vi "Distance PWM-Read.vi"(8 "Error":errorcluster, 11 "SonarMB1010DigitalDevRef":T1={"CounterDevRef"={"DevStatus"={"status"=FALSE, "code"=0, "source"=""}, "CntIndex"=enum."Invalid"}, "Min Distance"=0.000147, "Max Distance"=0.000147, "PWM Frequency"=0.0, "DIO Channel"=enum."DIO 0"}) -> (0 "Error Out":errorcluster, 2 "Distance Out":dbl, 3 "SonarMB1010DigitalDevRef Out":T1={"CounterDevRef"={"DevStatus"={"status"=FALSE, "code"=0, "source"=""}, "CntIndex"=enum."Invalid"}, "Min Distance"=0.000147, "Max Distance"=0.000147, "PWM Frequency"=0.0, "DIO Channel"=enum."DIO 0"})   [LabVIEW 2017]
doc: "Returns the distance, in inches, between the ultrasonic sensor and the closest object in front of the sensor. The ultrasonic sensor measures this distance by emitting a ping and calculating the time it takes for the echo of the ping to return. If the ultrasonic sensor does not detect the echo of the ping in 50 ms or less, the VI times out and returns a <B>Distance</B> value of 0."
uses:
  TypeDefs Distance/Cluster_Distance PWM Reference.ctl
  <vilib>/Rock Robotics/WPI/Counter/WPI_CounterDevRef.ctl
  <vilib>/Rock Robotics/SystemInterfaces/Counter/FPGA_CounterCtrSystemIndex.ctl
  <vilib>/Rock Robotics/SystemInterfaces/DIO/FPGA_DIOChannel.ctl
  <vilib>/Rock Robotics/WPI/DigitalModule/WPI_DigitalModuleDeviceRef.ctl
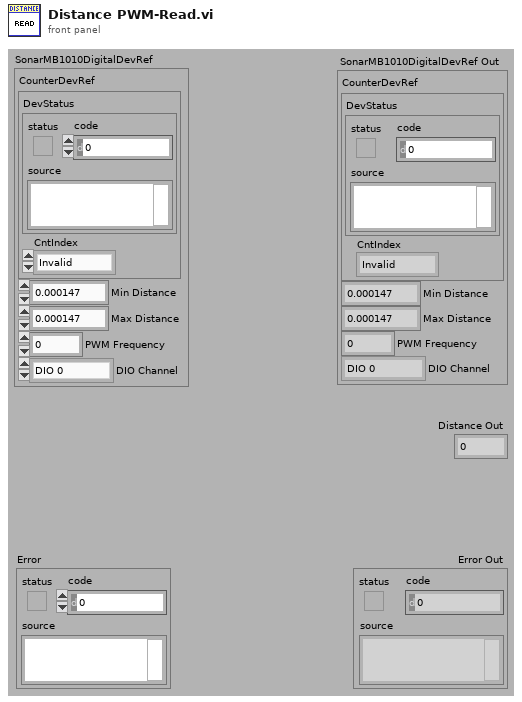
[diagram p1: front panel]
types:
  T1 = typedef "Cluster_Distance PWM Reference.ctl" = cluster{"CounterDevRef":T2, "Min Distance":dbl, "Max Distance":dbl, "PWM Frequency":dbl, "DIO Channel":T4}
  T2 = typedef "WPI_CounterDevRef.ctl" = cluster{"DevStatus":errorcluster, "CntIndex":T3}
  T3 = typedef "FPGA_CounterCtrSystemIndex.ctl" = enum8{"Ctr 0", "Ctr 1", "Ctr 2", "Ctr 3", "Ctr 4", "Ctr 5", "Ctr 6", "Ctr 7", "Invalid"}
  T4 = typedef "FPGA_DIOChannel.ctl" = enum8{"DIO 0", "DIO 1", "DIO 2", "DIO 3", "DIO 4", "DIO 5", "DIO 6", "DIO 7", "DIO 8", "DIO 9", "DIO MXP 0", "DIO MXP 1", "DIO MXP 2", "DIO MXP 3", "DIO MXP 4", "DIO MXP 5", "DIO MXP 6", "DIO MXP 7", "DIO MXP 8", "DIO MXP 9", "DIO MXP 10", "DIO MXP 11", "DIO MXP 12", "DIO MXP 13", "DIO MXP 14", "DIO MXP 15", "SPI Port CS1", "SPI Port CS2", "SPI Port CS3", "SPI Port MISO", "SPI Port MOSI", "Invalid"}
  T5 = typedef "WPI_DigitalModuleDeviceRef.ctl" = cluster{"DevStatus":errorcluster}
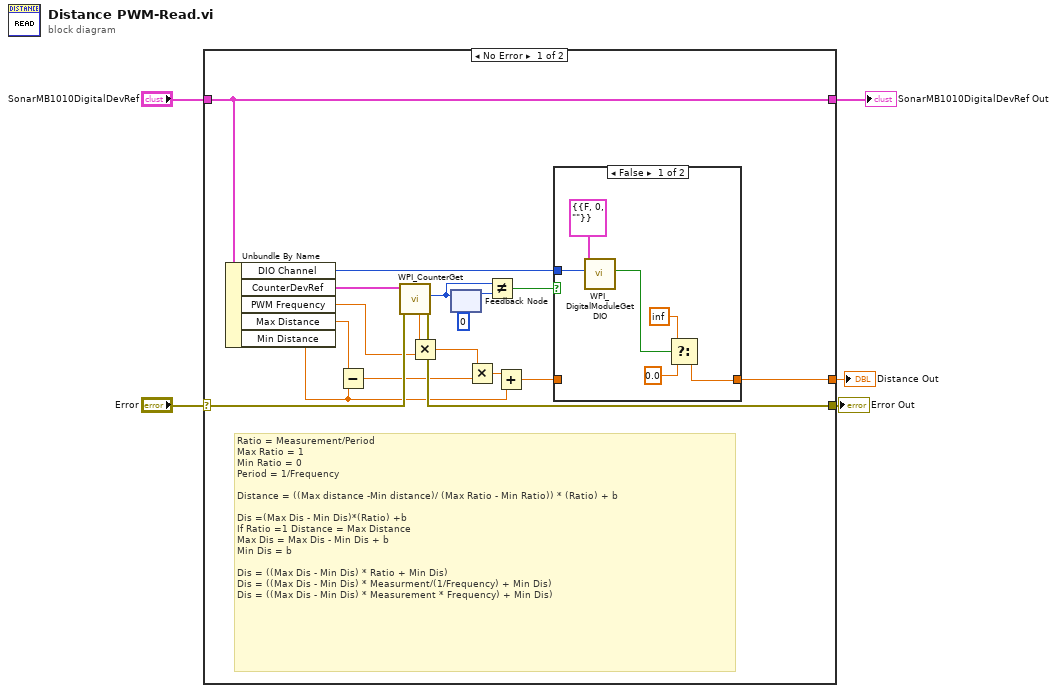
[diagram p0: block diagram]
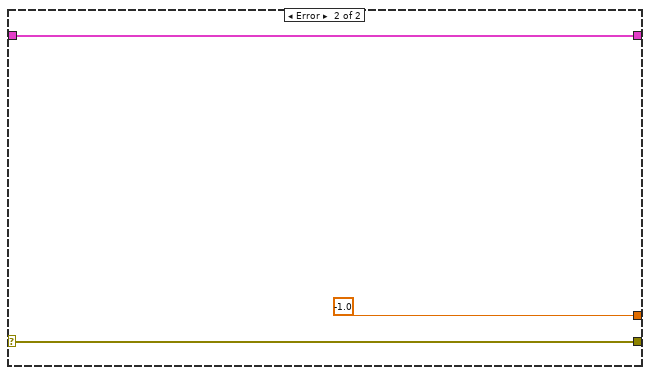
[diagram p3: hidden frame]
diagram:
  n1 = case shown="No Error" "Error" {
    selector: "Error" -> [w22 w33]
    tunnel: "SonarMB1010DigitalDevRef" -> [w20 w32]
    tunnel: [w20 w32] -> w1
    tunnel: [w21 w33] -> w5
    tunnel: [w6 -1.0] -> w3
    frame No Error {
      # "Ratio = Measurement/Period\nMax Ratio = 1\nMin Ratio = 0\nPeriod = 1/Frequency\n\nDistance = ((Max distance -Min distance)/ (Max Ratio - Min Ratio)) * (Ratio) + b\n\nDis =(Max Dis - Min Dis)*(Ratio) +b\nIf Ratio =1 Distance = Max Distance\nMax Dis = Max Dis - Min Dis + b\nMin Dis = b\n\nDis = ((Max Dis - Min Dis) * Ratio + Min Dis)\nDis = ((Max Dis - Min Dis) * Measurment/(1/Frequency) + Min Dis)\nDis = ((Max Dis - Min Dis) * Measurement * Frequency) + Min Dis)"
      n2 = Unbundle By Name(w20) -> ("DIO Channel"=w8:T4, "CounterDevRef"=w23:T2, "PWM Frequency"=w10:dbl, "Max Distance"=w18:dbl, "Min Distance"=w14:dbl)
      n3 = Subtract(x=w18, y=w14) -> (x-y=w16:dbl)
      n4 = call <vilib>:"WPI_CounterGet.vi"("error in (no error)"=w22, "CounterDevRef in"=w23) -> ("error out"=w21:errorcluster, "Value"=w12:i32, "Period (sec)"=w19:dbl)  [unwired: 4 in, 3 out]
      n5 = Multiply(x=w19, y=w10) -> (x*y=w17:dbl)
      n6 = feedback #1(0 ("Value")) -> (w13:i32)
      n7 = feedback-in #1(w12) -> ()
      n8 = Multiply(x=w17, y=w16) -> (x*y=w15:dbl)
      n9 = Not Equal?(x=w12, y=w13) -> (x != y?=w9:bool)
      n10 = Add(x=w15, y=w14) -> (x+y=w7:dbl)
      n11 = case shown="False" w9 {
        tunnel: w8 -> [w28 _]
        tunnel: w7 -> [_ w30]
        tunnel: [w24 w30] -> w6
        frame False {
          n12 = call <vilib>:"WPI_DigitalModuleGetDIO.vi"("DIOChannel"=w28, "DigitalModuleDevRef"=T5 {"DevStatus"={"status"=FALSE, "code"=0, "source"=""}}) -> ("Value"=w27:bool)  [unwired: 1 in, 8 out]
          n13 = Select(t=inf, s=w27, f=0.0 ("t")) -> (s? t:f=w24:dbl)
        }
        frame True {
        }
      }
    }
    frame Error {
    }
  }
  "Error Out" <- w5
  "Distance Out" <- w3
  "SonarMB1010DigitalDevRef Out" <- w1
